vi "Swerve steering init.vi"(8 "error in (no error)":errorcluster, 9 "timeoutMs":u32=100, 11 "PhoenixMotorControlDevRef In":T1={"DeviceStatus"={"status"=FALSE, "code"=0, "source"=""}, "Type"=enum."PWM", "PWM"={"PWM Channel"=enum."PWM 1", "DeadBand"={"Name"="", "maxPositivePwm"=0, "minPositivePwm"=0, "centerPwm"=0, "maxNegativePwm"=0, "minNegativePwm"=0, "angularRange"=0}}, "CAN"={"Device Number"=0, "SetOutput VI Ref"=variant(enum8{"Percent VBus", "Current", "Speed", "Position", "Voltage"} enum."Percent VBus"), "GetOutput VI Ref"=variant(refnum<k1> refnum), "Enable VI Ref"=variant(dbl 12.0), "Disable VI Ref"=variant(enum8{"Percent VBus", "Speed", "Position", "Slave", "Unchanged / Invalid", "Voltage Compensation", "Current", "Motion Profile"} enum."Percent VBus"), "Data"=variant}, "Invert"=FALSE, "DIO PWM"={"PWM \"Enable\" Channel"=enum."Invalid", "DIOChannel"=enum."Invalid", "PWM Rate"=0.0}}) -> (0 "error out":errorcluster, 3 "PhoenixMotorControlDevRef Out":T1={"DeviceStatus"={"status"=FALSE, "code"=0, "source"=""}, "Type"=enum."PWM", "PWM"={"PWM Channel"=enum."PWM 1", "DeadBand"={"Name"="", "maxPositivePwm"=0, "minPositivePwm"=0, "centerPwm"=0, "maxNegativePwm"=0, "minNegativePwm"=0, "angularRange"=0}}, "CAN"={"Device Number"=0, "SetOutput VI Ref"=variant(enum8{"Percent VBus", "Current", "Speed", "Position", "Voltage"} enum."Percent VBus"), "GetOutput VI Ref"=variant(refnum<k1> refnum), "Enable VI Ref"=variant(dbl 12.0), "Disable VI Ref"=variant(enum8{"Percent VBus", "Speed", "Position", "Slave", "Unchanged / Invalid", "Voltage Compensation", "Current", "Motion Profile"} enum."Percent VBus"), "Data"=variant}, "Invert"=FALSE, "DIO PWM"={"PWM \"Enable\" Channel"=enum."Invalid", "DIOChannel"=enum."Invalid", "PWM Rate"=0.0}})   [LabVIEW 2018]
uses:
  <vilib>/Rock Robotics/WPI/MotorControl/WPI_MotorControlDeviceRef.ctl
  <vilib>/Rock Robotics/WPI/MotorControl/WPI_MotorControlType.ctl
  <vilib>/Rock Robotics/SystemInterfaces/DIO/FPGA_DIOPWMChannel.ctl
  <vilib>/Rock Robotics/WPI/PWM/WPI_PWMDeadband.ctl
  <vilib>/Rock Robotics/SystemInterfaces/DIO/FPGA_DIOChannel.ctl
  <vilib>/Rock Robotics/WPI/ThirdParty/Phoenix-LabVIEW/Motor Controller/Controls/CTRE_Phoenix_MotorControl_FeedbackDevice.ctl
  <vilib>/Rock Robotics/WPI/ThirdParty/Phoenix-LabVIEW/Motor Controller/Controls/CTRE_Phoenix_MotorControl_NeutralMode.ctl
panel:
  in  "F":dbl
  in  "D":dbl
  in  "I":dbl
  in  "P":dbl=10.0
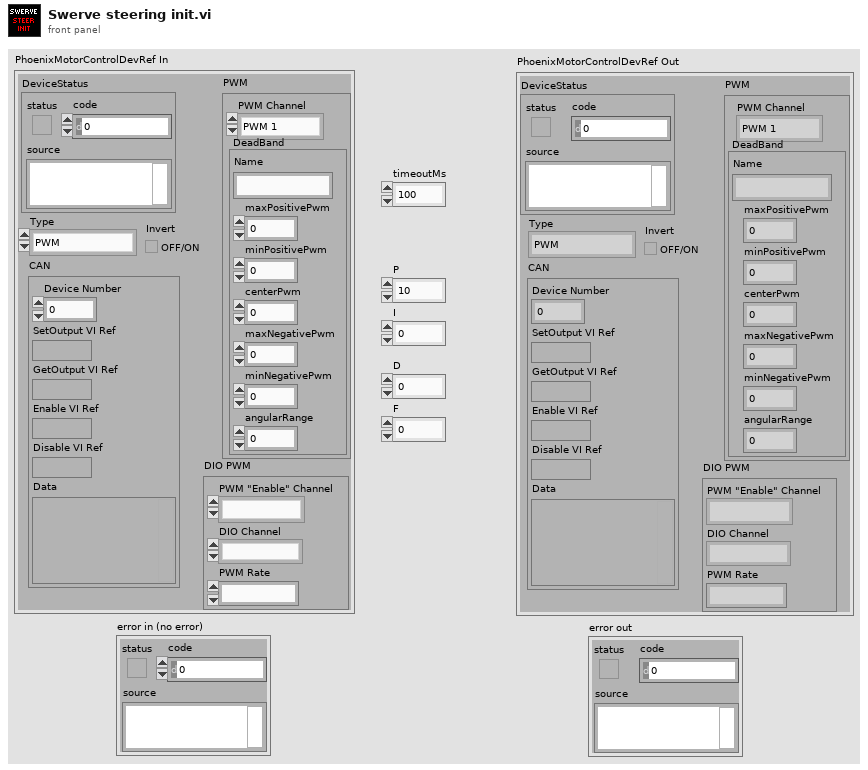
[diagram p1: front panel]
types:
  T1 = typedef "WPI_MotorControlDeviceRef.ctl" = cluster{"DeviceStatus":errorcluster, "Type":T2, "PWM":cluster{"PWM Channel":T3, "DeadBand":T4}, "CAN":cluster{"Device Number":u8, "SetOutput VI Ref":variant, "GetOutput VI Ref":variant, "Enable VI Ref":variant, "Disable VI Ref":variant, "Data":variant}, "Invert":bool, "DIO PWM":cluster{"PWM \"Enable\" Channel":T3, "DIOChannel":T5, "PWM Rate":dbl}}
  T2 = typedef "WPI_MotorControlType.ctl" = enum16{"PWM", "CAN", "DIO PWM"}
  T3 = typedef "FPGA_DIOPWMChannel.ctl" = enum8{"PWM 0", "PWM 1", "PWM 2", "PWM 3", "PWM 4", "PWM 5", "PWM 6", "PWM 7", "PWM 8", "PWM 9", "PWM MXP 0", "PWM MXP 1", "PWM MXP 2", "PWM MXP 3", "PWM MXP 4", "PWM MXP 5", "PWM MXP 6", "PWM MXP 7", "PWM MXP 8", "PWM MXP 9", "Invalid"}
  T4 = typedef "WPI_PWMDeadband.ctl" = cluster{"Name":string, "maxPositivePwm":i32, "minPositivePwm":i32, "centerPwm":i32, "maxNegativePwm":i32, "minNegativePwm":i32, "angularRange":u16}
  T5 = typedef "FPGA_DIOChannel.ctl" = enum8{"DIO 0", "DIO 1", "DIO 2", "DIO 3", "DIO 4", "DIO 5", "DIO 6", "DIO 7", "DIO 8", "DIO 9", "DIO MXP 0", "DIO MXP 1", "DIO MXP 2", "DIO MXP 3", "DIO MXP 4", "DIO MXP 5", "DIO MXP 6", "DIO MXP 7", "DIO MXP 8", "DIO MXP 9", "DIO MXP 10", "DIO MXP 11", "DIO MXP 12", "DIO MXP 13", "DIO MXP 14", "DIO MXP 15", "SPI Port CS1", "SPI Port CS2", "SPI Port CS3", "SPI Port MISO", "SPI Port MOSI", "Invalid"}
  T6 = typedef "CTRE_Phoenix_MotorControl_NeutralMode.ctl" = enum8{"EEPROMSetting", "Override to Coast", "Override to Brake"}
  T7 = typedef "CTRE_Phoenix_MotorControl_FeedbackDevice.ctl" = i8
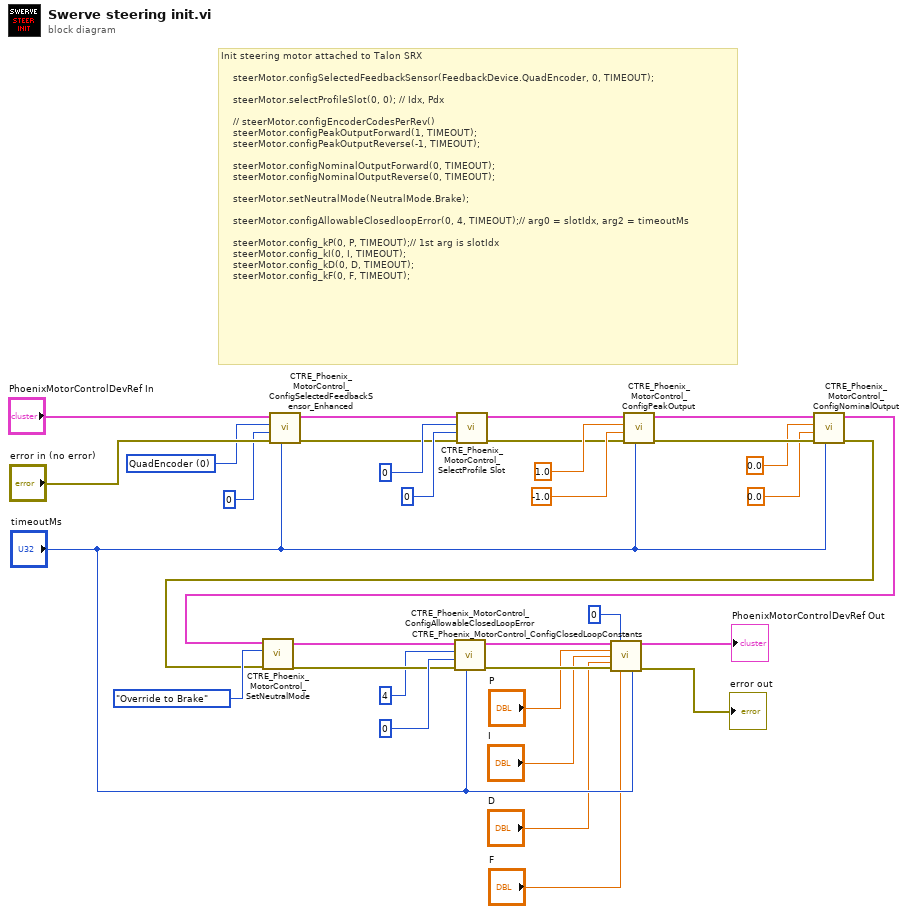
[diagram p0: block diagram]
diagram:
  w14 = T7 0 items=["QuadEncoder"=0, "Analog"=2, "Tachometer"=4, "Pulse Width Encoded Position"=8, "Sensor Sum (S0 + S1)"=9, "Sensor Difference (D0 - D1)"=10, "Remote Source 0"=11, "Remote Source 1"=12, "Software Emulated"=15] ("Feedback Device")
  # "Init steering motor attached to Talon SRX\n\n    steerMotor.configSelectedFeedbackSensor(FeedbackDevice.QuadEncoder, 0, TIMEOUT);\n\n    steerMotor.selectProfileSlot(0, 0); // Idx, Pdx\n\n    // steerMotor.configEncoderCodesPerRev()\n    steerMotor.configPeakOutputForward(1, TIMEOUT);\n    steerMotor.configPeakOutputReverse(-1, TIMEOUT);\n\n    steerMotor.configNominalOutputForward(0, TIMEOUT);\n    steerMotor.configNominalOutputReverse(0, TIMEOUT);\n\n    steerMotor.setNeutralMode(NeutralMode.Brake);\n\n    steerMotor.configAllowableClosedloopError(0, 4, TIMEOUT);// arg0 = slotIdx, arg2 = timeoutMs\n\n    steerMotor.config_kP(0, P, TIMEOUT);// 1st arg is slotIdx\n    steerMotor.config_kI(0, I, TIMEOUT);\n    steerMotor.config_kD(0, D, TIMEOUT);\n    steerMotor.config_kF(0, F, TIMEOUT);"
  n1 = call <vilib>:"CTRE_Phoenix_MotorControl_ConfigSelectedFeedbackSensor_Enhanced.vi"("timeoutMs"="timeoutMs", "error in (no error)"="error in (no error)", "pidLoopIdx"=0, "Feedback Device"=w14, "PhoenixMotorControlDevRef"="PhoenixMotorControlDevRef In") -> ("error out"=w18:errorcluster, "PhoenixMotorControlDevRef"=w19:T1)  [unwired: 5 in]
  n2 = call <vilib>:"CTRE_Phoenix_MotorControl_SelectProfile Slot.vi"("error in (no error)"=w18, "pidLoopIdx"=0, "slotIdx"=0, "PhoenixMotorControlDevRef"=w19) -> ("error out"=w22:errorcluster, "PhoenixMotorControlDevRef"=w23:T1)  [unwired: 6 in]
  n3 = call <vilib>:"CTRE_Phoenix_MotorControl_ConfigPeakOutput.vi"("timeoutMs"="timeoutMs", "error in (no error)"=w22, "Reverse Peak Percent Output"=-1.0, "Forward Peak Percent Output"=1.0, "PhoenixMotorControlDevRef"=w23) -> ("error out"=w29:errorcluster, "PhoenixMotorControlDevRef"=w28:T1)  [unwired: 5 in]
  n4 = call <vilib>:"CTRE_Phoenix_MotorControl_ConfigNominalOutput.vi"("timeoutMs"="timeoutMs", "error in (no error)"=w29, "Reverse Nominal Percent Output"=0.0, "Forward Nominal Percent Output"=0.0, "PhoenixMotorControlDevRef"=w28) -> ("error out"=w10:errorcluster, "PhoenixMotorControlDevRef"=w9:T1)  [unwired: 5 in]
  n5 = call <vilib>:"CTRE_Phoenix_MotorControl_SetNeutralMode.vi"("error in (no error)"=w10, "Motor Control Neutral Mode"=CTRE_Phoenix_MotorControl_NeutralMode."Override to Brake", "PhoenixMotorControlDevRef"=w9) -> ("error out"=w12:errorcluster, "PhoenixMotorControlDevRef"=w13:T1)  [unwired: 7 in]
  n6 = call <vilib>:"CTRE_Phoenix_MotorControl_ConfigAllowableClosedLoopError.vi"("timeoutMs"="timeoutMs", "error in (no error)"=w12, "slotIdx"=u32 0, "allowableClosedLoopError"=4, "PhoenixMotorControlDevRef"=w13) -> ("error out"=w30:errorcluster, "PhoenixMotorControlDevRef"=w31:T1)  [unwired: 5 in]
  n7 = call <vilib>:"CTRE_Phoenix_MotorControl_ConfigClosedLoopConstants.vi"("PhoenixMotorControlDevRef"=w31, "slotIdx"=0, "P"="P", "I"="I", "D"="D", "error in (no error)"=w30, "F"="F", "timeoutMs"="timeoutMs") -> ("PhoenixMotorControlDevRef"=→"PhoenixMotorControlDevRef Out":T1, "error out"=→"error out":errorcluster)  [unwired: 6 in]
